vi "Climb Control Loop.vi"() -> ()   [LabVIEW 2019]
uses:
  Calculations or utilities/Is command done typedef.ctl
  <vilib>/Rock Robotics/WPI/ThirdParty/Phoenix-LabVIEW/Motor Controller/Controls/CTRE_Phoenix_MotorControl_ControlMode.ctl
  Climb Global.vi
  <vilib>/Rock Robotics/WPI/ThirdParty/Phoenix-LabVIEW/Motor Controller/Get/CTRE_Phoenix_MotorController_GetLimitSwitchStates.vi
panel:
  out "Reverse Limit Closed?":bool
  out "Forward Limit Closed?":bool
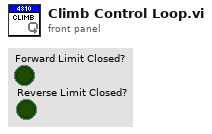
[diagram p1: front panel]
types:
  T1 = typedef "WPI_MotorControlDeviceRef.ctl" = cluster{"DeviceStatus":errorcluster, "Type":T2, "PWM":cluster{"PWM Channel":T3, "DeadBand":T4}, "CAN":cluster{"Device Number":u8, "SetOutput VI Ref":variant, "GetOutput VI Ref":variant, "Enable VI Ref":variant, "Disable VI Ref":variant, "Data":variant}, "Invert":bool, "DIO PWM":cluster{"PWM \"Enable\" Channel":T3, "DIOChannel":T5, "PWM Rate":dbl}}
  T2 = typedef "WPI_MotorControlType.ctl" = enum16{"PWM", "CAN", "DIO PWM"}
  T3 = typedef "FPGA_DIOPWMChannel.ctl" = enum8{"PWM 0", "PWM 1", "PWM 2", "PWM 3", "PWM 4", "PWM 5", "PWM 6", "PWM 7", "PWM 8", "PWM 9", "PWM MXP 0", "PWM MXP 1", "PWM MXP 2", "PWM MXP 3", "PWM MXP 4", "PWM MXP 5", "PWM MXP 6", "PWM MXP 7", "PWM MXP 8", "PWM MXP 9", "Invalid"}
  T4 = typedef "WPI_PWMDeadband.ctl" = cluster{"Name":string, "maxPositivePwm":i32, "minPositivePwm":i32, "centerPwm":i32, "maxNegativePwm":i32, "minNegativePwm":i32, "angularRange":u16}
  T5 = typedef "FPGA_DIOChannel.ctl" = enum8{"DIO 0", "DIO 1", "DIO 2", "DIO 3", "DIO 4", "DIO 5", "DIO 6", "DIO 7", "DIO 8", "DIO 9", "DIO MXP 0", "DIO MXP 1", "DIO MXP 2", "DIO MXP 3", "DIO MXP 4", "DIO MXP 5", "DIO MXP 6", "DIO MXP 7", "DIO MXP 8", "DIO MXP 9", "DIO MXP 10", "DIO MXP 11", "DIO MXP 12", "DIO MXP 13", "DIO MXP 14", "DIO MXP 15", "SPI Port CS1", "SPI Port CS2", "SPI Port CS3", "SPI Port MISO", "SPI Port MOSI", "Invalid"}
  T6 = typedef "Is command done typedef.ctl" = cluster{"Done?":bool, "Timestamp [ms]":dbl}
  T7 = typedef "Climb Command Type Def.ctl" = cluster{"Climb Mode":T8, "Throttle (%)":dbl, "Timestamp (ms)":dbl, "Skywalker Throttle (%)":dbl, " Climb Hook Throttle (%)":dbl}
  T8 = typedef "Climb Mode Type Def.ctl" = enum16{"Disabled", "Raw Throttle"}
  T9 = typedef "CTRE_Phoenix_MotorControl_ControlMode.ctl" = u16
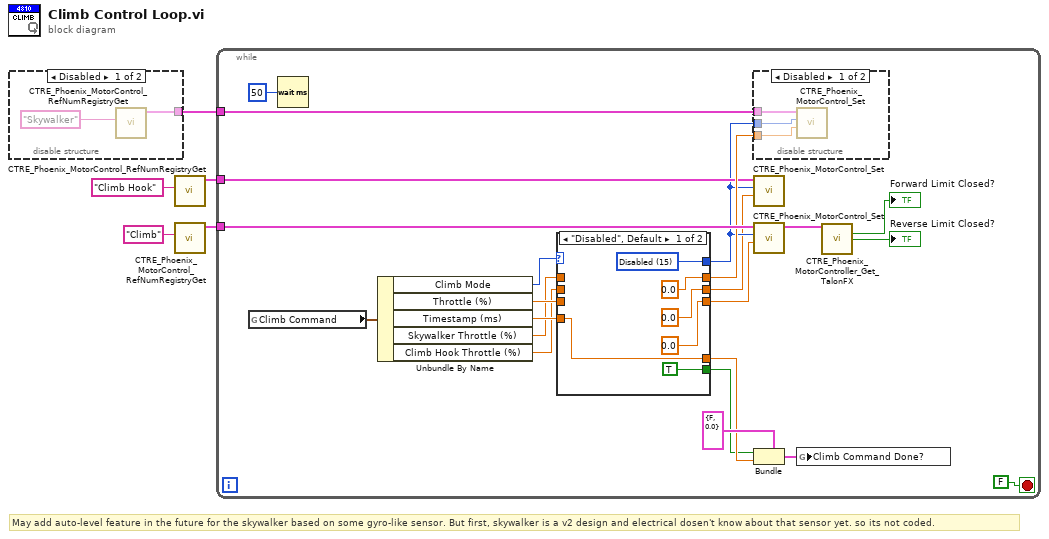
[diagram p0: block diagram]
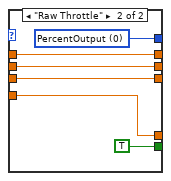
[diagram p4: hidden frame]
diagram:
  # "May add auto-level feature in the future for the skywalker based on some gyro-like sensor. But first, skywalker is a v2 design and electrical dosen't know about that sensor yet. so its not coded."
  n1 = disable-structure shown="Disabled" {
    disable-tunnel: [w6 _] -> w3
    frame Disabled {
      n2 = call <vilib>:"CTRE_Phoenix_MotorControl_RefNumRegistryGet.vi"("refnum name"="Skywalker") -> ("PhoenixMotorControlDevRef"=w6:T1)  [unwired: 9 in, 1 out]
    }
    frame Enabled {
    }
  }
  n3 = call <vilib>:"CTRE_Phoenix_MotorControl_RefNumRegistryGet.vi"("refnum name"="Climb Hook") -> ("PhoenixMotorControlDevRef"=w1:T1)  [unwired: 9 in, 1 out]
  n4 = call <vilib>:"CTRE_Phoenix_MotorControl_RefNumRegistryGet.vi"("refnum name"="Climb") -> ("PhoenixMotorControlDevRef"=w4:T1)  [unwired: 9 in, 1 out]
  n5 = while {
    tunnel: w4 -> [w27]
    tunnel: w3 -> [w17]
    tunnel: w1 -> [w11]
    stop <- FALSE stop-if-true
    n6 = global read "Climb Global.vi" "Climb Command"() -> (w18:T7)
    n7 = Wait (ms)(milliseconds to wait=u32 50) -> ()  [unwired: 1 out]
    n8 = Unbundle By Name(w18) -> ("Climb Mode"=w26:T8, "Throttle (%)"=w23:dbl, "Timestamp (ms)"=w25:dbl, "Skywalker Throttle (%)"=w13:dbl, "Climb Hook Throttle (%)"=w9:dbl)
    n9 = case shown="\"Disabled\", Default" w26 {
      tunnel: [w38 w42] -> w10
      tunnel: [w37 w43] -> w21
      tunnel: w25 -> [w37 w43]
      tunnel: [0.0 ("Throttle (%)") w44] -> w24
      tunnel: w23 -> [_ w44]
      tunnel: [TRUE ("Done?") TRUE ("Done?")] -> w20
      tunnel: w13 -> [_ w40]
      tunnel: [0.0 ("Skywalker Throttle (%)") w40] -> w12
      tunnel: w9 -> [_ w39]
      tunnel: [0.0 ("Climb Hook Throttle (%)") w39] -> w8
      frame "Disabled", Default {
        w38 = T9 15 items=["PercentOutput"=0, "Position"=1, "Velocity"=2, "Current"=3, "Follower"=5, "MotionProfile"=6, "MotionMagic"=7, "MotionProfileArc"=10, "Disabled"=15] ("Control Mode")
      }
      frame "Raw Throttle" {
        w42 = T9 0 items=["PercentOutput"=0, "Position"=1, "Velocity"=2, "Current"=3, "Follower"=5, "MotionProfile"=6, "MotionMagic"=7, "MotionProfileArc"=10, "Disabled"=15] ("Control Mode")
      }
    }
    n10 = disable-structure shown="Disabled" {
      disable-tunnel: w17 -> [w32 _]
      disable-tunnel: w12 -> [w31 _]
      disable-tunnel: w10 -> [w30 _]
      frame Disabled {
        n11 = call <vilib>:"CTRE_Phoenix_MotorControl_Set.vi"("Output"=w31, "Control Mode"=w30, "PhoenixMotorControlDevRef"=w32) -> ()  [unwired: 7 in, 2 out]
      }
      frame Enabled {
      }
    }
    n12 = call <vilib>:"CTRE_Phoenix_MotorControl_Set.vi"("Output"=w8, "Control Mode"=w10, "PhoenixMotorControlDevRef"=w11) -> ()  [unwired: 7 in, 2 out]
    n13 = call <vilib>:"CTRE_Phoenix_MotorControl_Set.vi"("Output"=w24, "Control Mode"=w10, "PhoenixMotorControlDevRef"=w27) -> ("PhoenixMotorControlDevRef"=w16:T1)  [unwired: 7 in, 1 out]
    n14 = Bundle(cluster=T6 {"Done?"=FALSE, "Timestamp [ms]"=0.0} ("Command Done?"), "Done?"=w20, "Timestamp [ms]"=w21) -> (w19:T6)
    n15 = global write "Climb Global.vi" "Climb Command Done?"(w19) -> ()
    n16 = call-poly <vilib>:"CTRE_Phoenix_MotorController_Get_TalonFX.vi"("PhoenixMotorControlDevRef"=w16) -> ("Forward Limit Closed?"=→"Forward Limit Closed?":bool, "Reverse Limit Closed?"=→"Reverse Limit Closed?":bool)  [unwired: 11 in, 2 out]
  }
